vi "example_2_5_a.vi"() -> ()   [LabVIEW 2018]
panel:
  out "Array":string[](array[string])
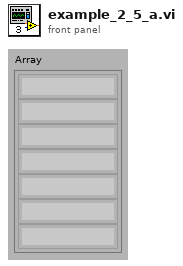
[diagram p1: front panel]
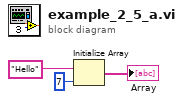
[diagram p0: block diagram]
diagram:
  n1 = Initialize Array("Hello", 7 ("Dimension Size")) -> (→"Array":string[])
